vi "Websocket Server Main.vi"(8 "Error In":errorcluster) -> (0 "Error Out":errorcluster)   [LabVIEW 2014]
uses:
  Controls/TCP State Machine States.ctl
  Globals/messages.vi
  Controls/TCP State Machine Data.ctl
  Globals/applicaiton-globals.vi
  <vilib>/MediaMongrels Ltd/WebSockets/WebSockets/WebSockets.lvlib
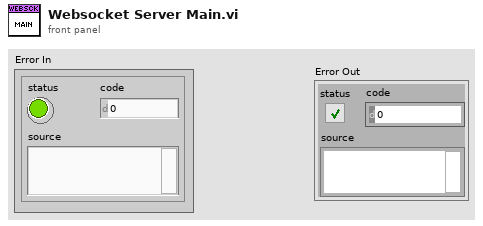
[diagram p1: front panel]
types:
  T1 = typedef "TCP State Machine Data.ctl" = cluster{"Clients":refnum<k5>[], "Listener":refnum<k5>}
  T2 = typedef "TCP State Machine States.ctl" = enum16{"Initialize", "Status Check", "Read Data", "Stop"}
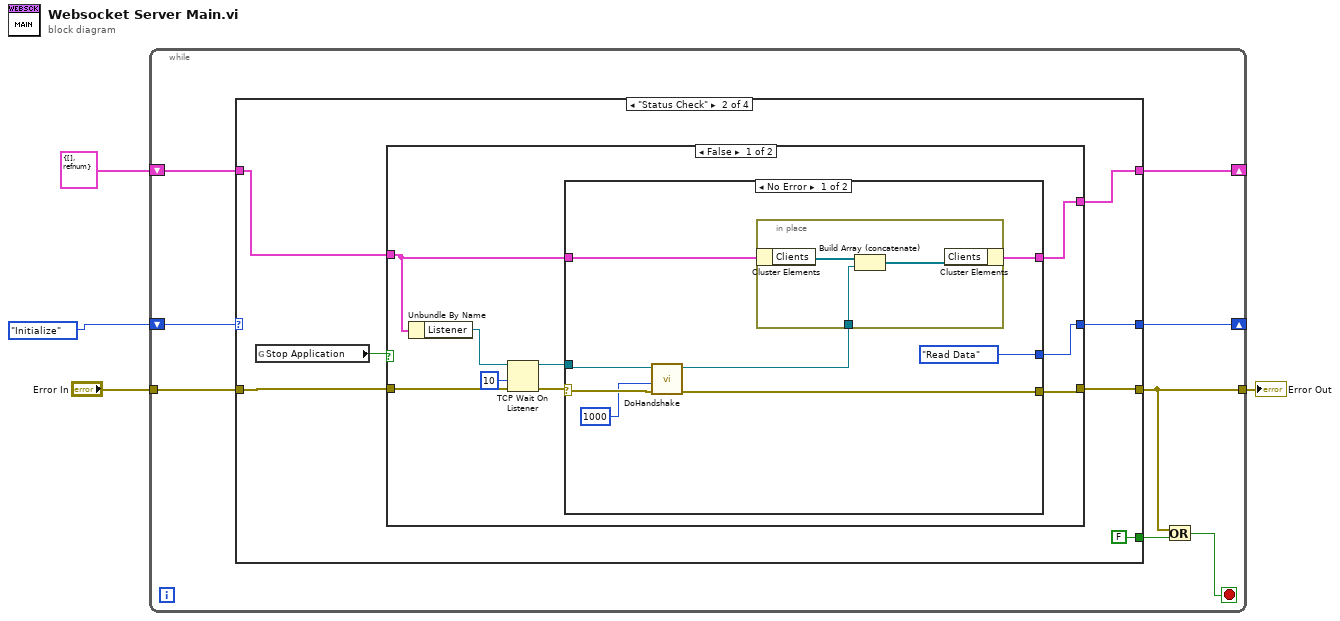
[diagram p0: block diagram]
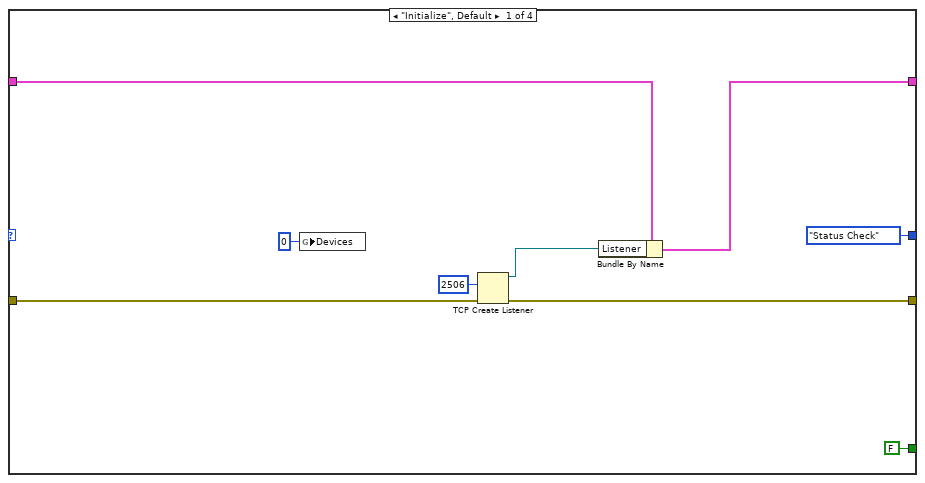
[diagram p2: hidden frame]
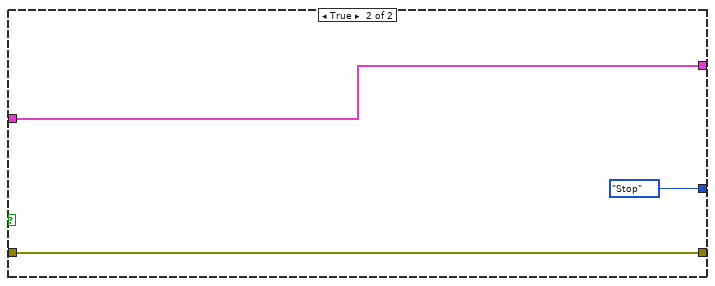
[diagram p4: hidden frame]
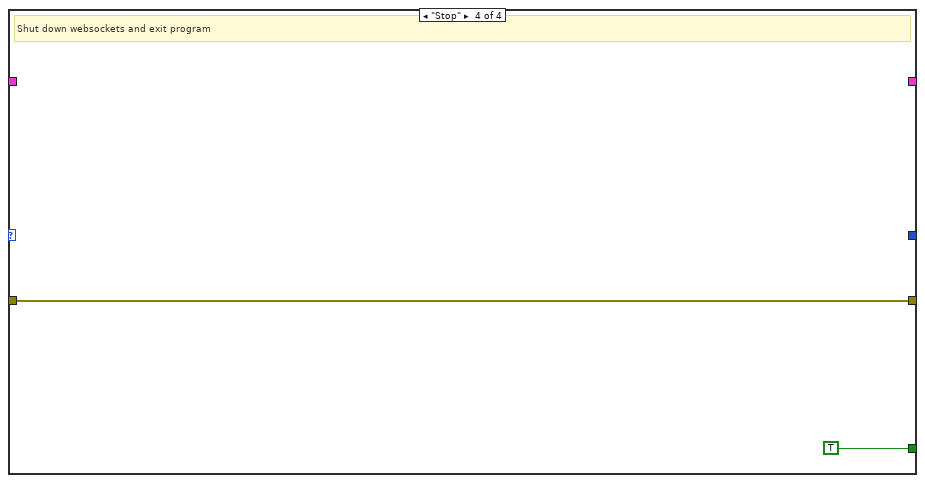
[diagram p6: hidden frame]
diagram:
  n1 = while {
    tunnel: "Error In" -> [w12]
    tunnel: [w8] -> w2
    shift-right: [w7] -> _
    shift-left: T1 {"Clients"=[], "Listener"=refnum} ("Data") -> [w6]
    shift-right: [w5] -> _
    shift-left: TCP_State_Machine_States."Initialize" ("States") -> [w11]
    stop <- w9 stop-if-true
    n2 = case shown="\"Status Check\"" w11 {
      tunnel: w12 -> [w20 w27 _ w52]
      tunnel: [FALSE FALSE _ TRUE] -> w10
      tunnel: [w19 w23 _ w52] -> w8
      tunnel: [w14 w25 _ _] -> w7
      tunnel: w6 -> [w16 w28 _ _]
      tunnel: [TCP_State_Machine_States."Status Check" ("States") w24 _ _] -> w5
      frame "Initialize", Default {
        n3 = global write "messages.vi" "Devices"(0 ("Devices")) -> ()
        n4 = TCP Create Listener(8:w20, 10:u16 2506 ("port")) -> (0:w19:errorcluster, 3:w15:refnum<k5>)  [unwired: 3 in, 1 out]
        n5 = Bundle By Name(cluster=w16, "Listener"=w15) -> (w14:T1)
      }
      frame "Status Check" {
        n6 = global read "applicaiton-globals.vi" "Stop Application"() -> (w26:bool)
        n7 = case shown="False" w26 {
          tunnel: w28 -> [w32 w51]
          tunnel: w27 -> [w37 w49]
          tunnel: [w31 w51] -> w25
          tunnel: [w29 TCP_State_Machine_States."Stop" ("States")] -> w24
          tunnel: [w30 w49] -> w23
          frame False {
            n8 = Unbundle By Name(w32) -> ("Listener"=w36:refnum<k5>)
            n9 = TCP Wait On Listener(8:w37, 9:10 ("timeout ms (wait forever: -1)"), 11:w36) -> (0:w34:errorcluster, 3:w33:refnum<k5>)  [unwired: 1 in, 3 out]
            n10 = case shown="No Error" w34 {
              selector: w34 -> [w45 _]
              tunnel: w33 -> [w44 _]
              tunnel: w32 -> [w42 _]
              tunnel: [w40 _] -> w31
              tunnel: [w39 _] -> w30
              tunnel: [TCP_State_Machine_States."Read Data" ("States") _] -> w29
              frame No Error {
                n11 = call <vilib>:"DoHandshake.vi"("error in (no error)"=w45, "timeout ms (5000)"=1000, "WebSocket Connection in"=w44) -> ("error out"=w39:errorcluster, "WebSocket Connection out"=w41:refnum<k5>)  [unwired: 5 in, 2 out]
                n12 = in-place {
                  in-place-border: w41 -> [w46]
                  n13 = in-place-cluster #1(w42) -> ("Clients"=w48:refnum<k5>[])
                  n14 = Build Array (concatenate)(w48, w46) -> (w47:refnum<k5>[])
                  n15 = in-place-cluster #1("Clients"=w47) -> (w40:T1)
                }
              }
              frame Error {
              }
            }
          }
          frame True {
            # "Application has been stopped. This is used for development running."
          }
        }
      }
      frame "Read Data" {
      }
      frame "Stop" {
        # "Shut down websockets and exit program"
      }
    }
    n16 = Or(x=w8, y=w10) -> (x .or. y?=w9:bool)
  }
  "Error Out" <- w2
